vi "Set Color by Name.vi"(8 "error in (no error)":errorcluster caption="错误输入（无错误）", 11 "name":string) -> (0 "error out":errorcluster caption="错误输出", 3 "FromName":refnum<k24>)   [LabVIEW 2012, in "Color.lvclass"]
uses:
  Color.lvclass
  System.Drawing
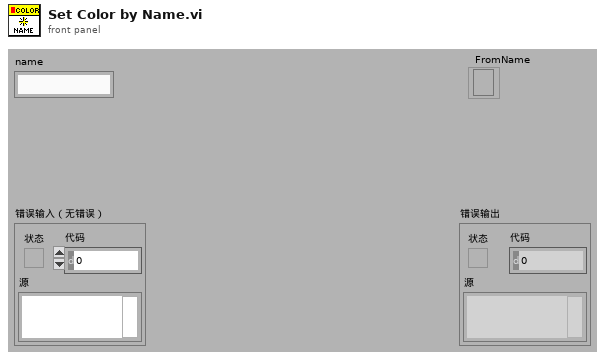
[diagram p1: front panel]
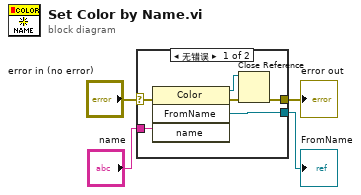
[diagram p0: block diagram]
diagram:
  n1 = case shown="无错误" "error in (no error)" {
    selector: "error in (no error)" -> [w10 w11]
    tunnel: [w9 w11] -> w3
    tunnel: "name" -> [w8 _]
    tunnel: [w5 _] -> w1
    frame No Error {
      n2 = invoke class="Color" method="FromName"(error in=w10, "name"=w8) -> (reference out=w7:refnum<k24>, error out=w6:errorcluster, "FromName"=w5:refnum<k24>)  [unwired: 2 in, 1 out]
      n3 = Close Reference(reference=w7, error in (no error)=w6) -> (error out=w9:errorcluster)
    }
    frame Error {
    }
  }
  "error out" <- w3
  "FromName" <- w1
